vi "EnaTrigTmstmp.vi"(8 "error in (no error)":errorcluster, 10 "clEnaTrigTmstmp":T1, 11 "SyncPluginBase in":refnum<class "SyncPluginBase.lvclass">) -> (0 "error out":errorcluster, 3 "SyncPluginBase out":refnum<class "SyncPluginBase.lvclass">)   [LabVIEW 2014, in "SyncPlugins.lvlib" / "SyncPluginBase.lvclass"]
uses:
  SyncPluginBase.lvclass
  Typedefs/clEnaTrigTmstmp.ctl
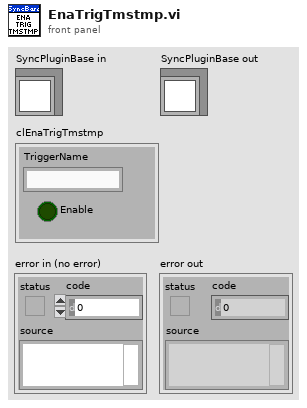
[diagram p1: front panel]
types:
  T1 = typedef "SyncPlugins.lvlib/SyncPluginBase.lvclass/clEnaTrigTmstmp.ctl" = cluster{"TriggerName":string, "Enable":bool}
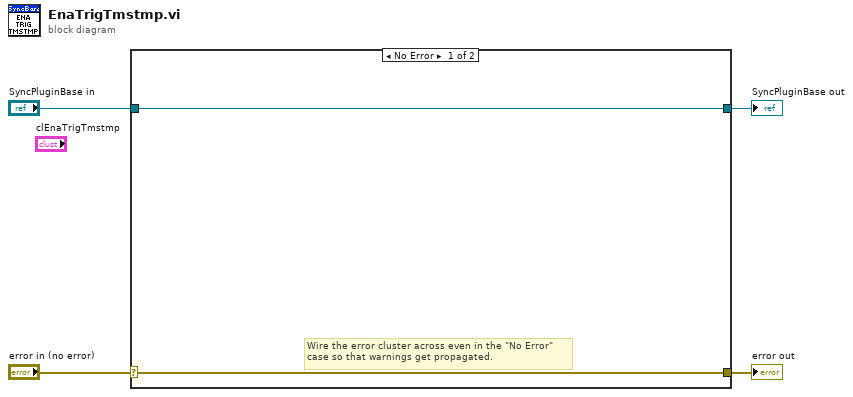
[diagram p0: block diagram]
diagram:
  n1 = case shown="No Error" "error in (no error)" {
    selector: "error in (no error)" -> [w5 w8]
    tunnel: [w5 w8] -> w3
    tunnel: [w6 w7] -> w1
    tunnel: "SyncPluginBase in" -> [w6 w7]
    frame No Error {
      # "Wire the error cluster across even in the \"No Error\"\ncase so that warnings get propagated."
    }
    frame Error {
    }
  }
  "error out" <- w3
  "SyncPluginBase out" <- w1
